vi "Write_Ch_data_file.vi"(4 "Append last row only":bool, 5 "Header string":string, 6 "Lock File":bool, 7 "exists?":bool, 8 "Write offset fr file end":i32, 9 "Channel Values":string[][](array[string]), 10 "Channel names":string[](array[string]), 11 "Filename":path) -> ()   [LabVIEW 2010]
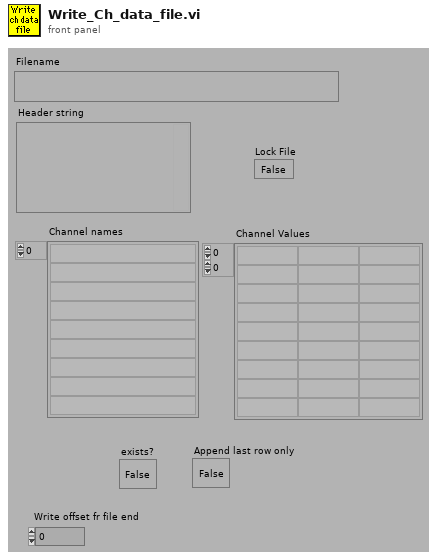
[diagram p1: front panel]
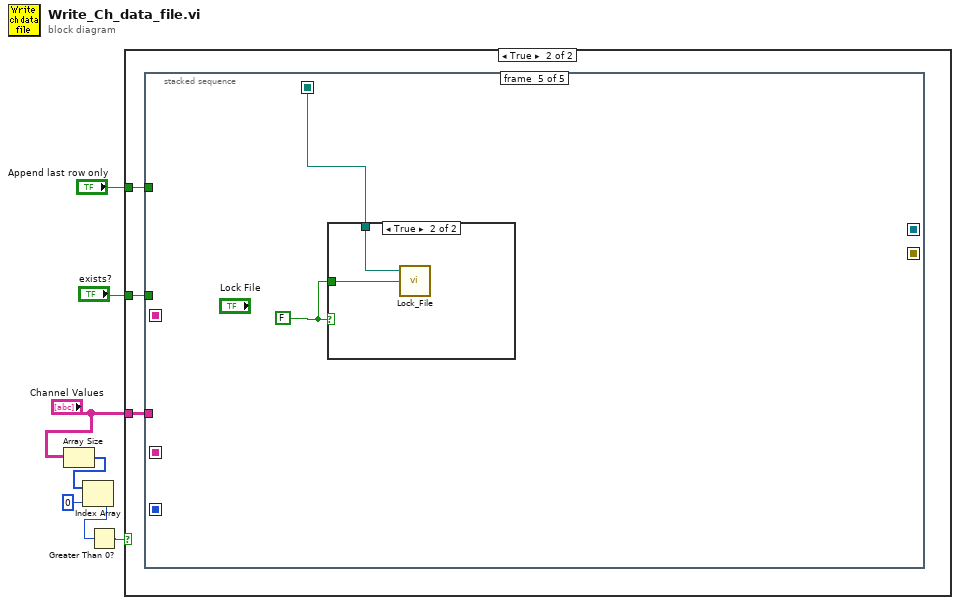
[diagram p0: block diagram]
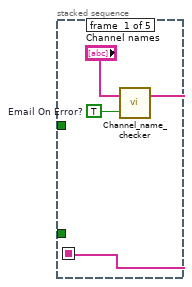
[diagram p3: hidden frame]
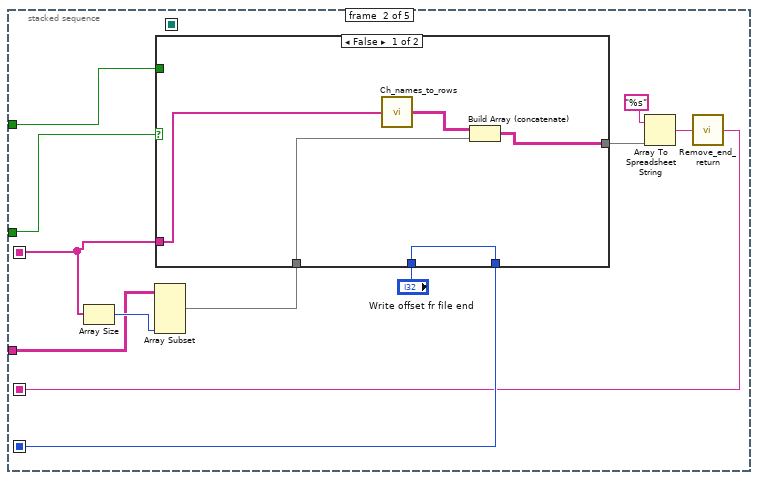
[diagram p4: hidden frame]
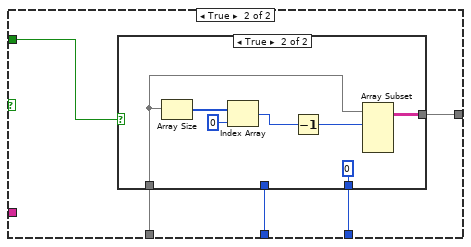
[diagram p5: hidden frame]
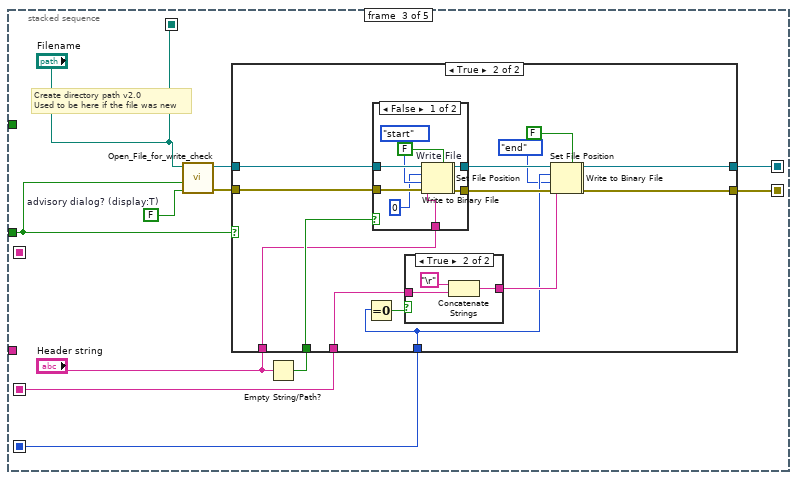
[diagram p7: hidden frame]
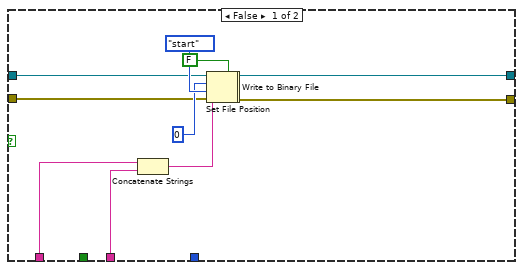
[diagram p8: hidden frame]
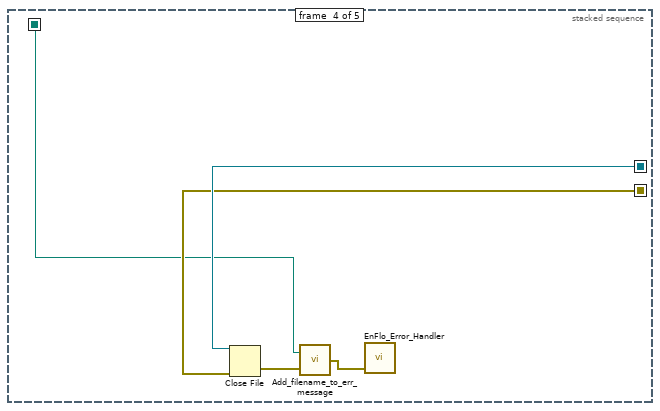
[diagram p11: hidden frame]
diagram:
  n1 = Array Size(array="Channel Values") -> (size(s)=w3:i32[])
  n2 = Index Array(array=w3, index=0 ("Index")) -> (element=w2:i32)
  n3 = Greater Than 0?(x=w2) -> (x > 0?=w1:bool)
  n4 = case shown="True" w1 {
    tunnel: "exists?" -> [_ w10]
    tunnel: "Append last row only" -> [_ w9]
    tunnel: "Channel Values" -> [_ w8]
    frame False {
    }
    frame True {
      n5 = stacked-sequence {
        seq-local: [_ w19 _ _ _] -> [_ _ w54 _ _]
        seq-local: [_ w22 _ _ _] -> [_ _ w51 _ _]
        seq-local: [_ _ w52 _ _] -> [_ _ _ w104 _]
        seq-local: [_ _ w50 _ _] -> [_ _ _ w103 _]
        seq-local: [w13 _ _ _ _] -> [_ w15 _ _ _]
        seq-local: [_ _ "Filename" _ _] -> [_ _ _ w101 w106]
        tunnel: w10 -> [_ w21 w46 _ _]
        tunnel: w9 -> [_ w23 _ _ _]
        tunnel: w8 -> [_ w16 _ _ _]
        frame #0 {
          w11 = TRUE  # Email On Error?
          n6 = call "Channel_name_checker.vi"("Email On Error?"=w11, "Channel names"="Channel names") -> ("Channel names Out"=w13:string[])  [unwired: 1 out]
        }
        frame #1 {
          n7 = Array Size(array=w15) -> (size(s)=w17:i32)
          n8 = Array Subset(array=w16, length (col)=w17) -> (w14:string[][])  [unwired: 3 in]
          n9 = case shown="False" w21 {
            tunnel: w15 -> [w27 _]
            tunnel: [w30 w32] -> w24
            tunnel: w23 -> [_ w35]
            tunnel: [w29 w34] -> w22
            tunnel: "Write offset fr file end" -> [w29 w33]
            tunnel: w14 -> [w26 w31]
            frame False {
              n10 = call "Ch_names_to_rows.vi"("Channel Names"=w27) -> ("3 Row names"=w28:string[][])
              n11 = Build Array (concatenate)(w28, w26) -> (w30:string[][])
            }
            frame True {
              n12 = case shown="True" w35 {
                tunnel: w31 -> [w37 w40]
                tunnel: [w37 w39] -> w32
                tunnel: [w36 0 ("Write offset fr file end")] -> w34
                tunnel: w33 -> [w36 _]
                frame False {
                }
                frame True {
                  n13 = Array Size(array=w40) -> (size(s)=w43:i32[])
                  n14 = Index Array(array=w43, index=0) -> (element=w41:i32)
                  n15 = Decrement(x=w41) -> (x-1=w42:i32)
                  n16 = Array Subset(array=w40, index (row)=w42) -> (w39:string[][])  [unwired: 3 in]
                }
              }
            }
          }
          n17 = Array To Spreadsheet String(array=w24, 3:"%s" ("format string")) -> (spreadsheet string=w20:string)  [unwired: 1 out]
          n18 = call "Remove_end_return.vi"("Input string"=w20) -> ("Output string"=w19:string)
        }
        frame #2 {
          w48 = FALSE  # advisory dialog? (display:T)
          # "Create directory path v2.0\nUsed to be here if the file was new"
          n19 = call "Open_File_for_write_check.vi"("advisory dialog? (display:T)"=w48, "append to file? (new file:F)"=w46, "file path"="Filename") -> ("error out"=w49:errorcluster, "refnum"=w47:refnum<file>)  [unwired: 7 out]
          n20 = Empty String/Path?(string/path="Header string") -> (empty?=w55:bool)
          n21 = case shown="True" w46 {
            tunnel: w55 -> [_ w81]
            tunnel: w51 -> [_ w74]
            tunnel: w54 -> [w63 w77]
            tunnel: [w65 w80] -> w50
            tunnel: "Header string" -> [w64 w79]
            tunnel: [w61 w78] -> w52
            tunnel: w47 -> [w60 w72]
            tunnel: w49 -> [w59 w73]
            frame False {
              n22 = Concatenate Strings(w64, w63) -> (w62:string)
              n23 = Set File Position(offset (in bytes) (0)=0 ("pos offset (0)"), refnum=w60, from (0:start)=enum16{"start", "end", "current"}."start" ("pos mode (0:2)"), error in=w59) -> (refnum out=w58:refnum<file>, error out=w57:errorcluster)
              n24 = Write to Binary File(file (use dialog)=w58, data=w62, error in=w57, 5:FALSE ("prepend array or string size? (T)")) -> (refnum out=w61:refnum<file>, error out=w65:errorcluster)  [unwired: 3 out]
            }
            frame True {
              n25 = Equal To 0?(x=w74) -> (x = 0?=w75:bool)
              n26 = case shown="False" w81 {
                tunnel: w72 -> [w97 w99]
                tunnel: w73 -> [w96 w98]
                tunnel: [w93 w99] -> w83
                tunnel: [w92 w98] -> w82
                tunnel: w79 -> [w91 _]
                frame False {
                  n27 = Set File Position(offset (in bytes) (0)=0 ("pos offset (0)"), refnum=w97, from (0:start)=enum16{"start", "end", "current"}."start" ("pos mode (0:2)"), error in=w96) -> (refnum out=w90:refnum<file>, error out=w89:errorcluster)
                  n28 = Write to Binary File "Write File"(file (use dialog)=w90, data=w91, error in=w89, 5:FALSE ("prepend array or string size? (T)")) -> (refnum out=w93:refnum<file>, error out=w92:errorcluster)  [unwired: 3 out]
                }
                frame True {
                }
              }
              n29 = case shown="True" w75 {
                tunnel: w77 -> [w84 w87]
                tunnel: [w84 w86] -> w76
                frame False {
                }
                frame True {
                  n30 = Concatenate Strings("\r", w87) -> (w86:string)
                }
              }
              n31 = Set File Position(offset (in bytes) (0)=w74, refnum=w83, from (0:start)=enum16{"start", "end", "current"}."end" ("pos mode (0:2)"), error in=w82) -> (refnum out=w70:refnum<file>, error out=w69:errorcluster)
              n32 = Write to Binary File(file (use dialog)=w70, data=w76, error in=w69, 5:FALSE ("prepend array or string size? (T)")) -> (refnum out=w78:refnum<file>, error out=w80:errorcluster)  [unwired: 3 out]
            }
          }
        }
        frame #3 {
          n33 = Close File(refnum=w104, error in=w103) -> (error out=w102:errorcluster)  [unwired: 1 out]
          n34 = call "Add_filename_to_err_message.vi"("error in (no error)"=w102, "Path"=w101) -> ("error out"=w100:errorcluster)
          n35 = call "EnFlo_Error_Handler.vi"("error in (no error)"=w100) -> ()  [unwired: 2 in, 3 out]
        }
        frame #4 {
          w105 = FALSE ("Lock File")
          n36 = case shown="True" w105 {
            tunnel: w105 -> [_ w108]
            tunnel: w106 -> [_ w107]
            frame False {
            }
            frame True {
              n37 = call "Lock_File.vi"("Lock File"=w108, "path"=w107) -> ()  [unwired: 1 in, 3 out]
            }
          }
        }
      }
    }
  }
